vi "Untitled 22.vi"() -> ()   [LabVIEW 2010]
uses:
  <vilib>/NXT/Block Support/NXT_InputPort.ctl
  <vilib>/NXT/Subs/MotorOutput.ctl
  <vilib>/NXT/Dual Mode Library/Sensors/Sonar_cm.vi
  <vilib>/NXT/Dual Mode Library/Motors/MotorOn.vi
  <vilib>/NXT/Dual Mode Library/Motors/MotorReverse.vi
  <vilib>/NXT/Dual Mode Library/Waits/Wait_Num.vi
panel:
  in  "Time (1 sec) 2":sgl=1.0 caption="Time (1 sec)"
  in  "Time (1 sec)":sgl=1.0
  in  "Output Port (All Ports) 2":T1=3 items=["Port A", "Port B", "Port C", "All Ports"]
  in  "Power (75)":i32=75
  in  "Output Port (All Ports)":T1=3 items=["Port A", "Port B", "Port C", "All Ports"]
  in  "Port (Port 4)":T2=3 items=["Port 1", "Port 2", "Port 3", "Port 4"]
  in  "stop":bool
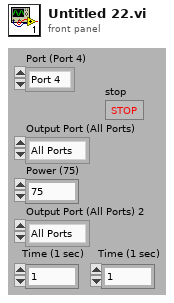
[diagram p1: front panel]
types:
  T1 = typedef "MotorOutput.ctl" = u8
  T2 = typedef "NXT_InputPort.ctl" = u8
  T3 = typedef "LVHSConnector.ctl" = cluster{"error":errorcluster, "address":string, "NXT #":i32, "Show Error":bool, "Connection":u16}
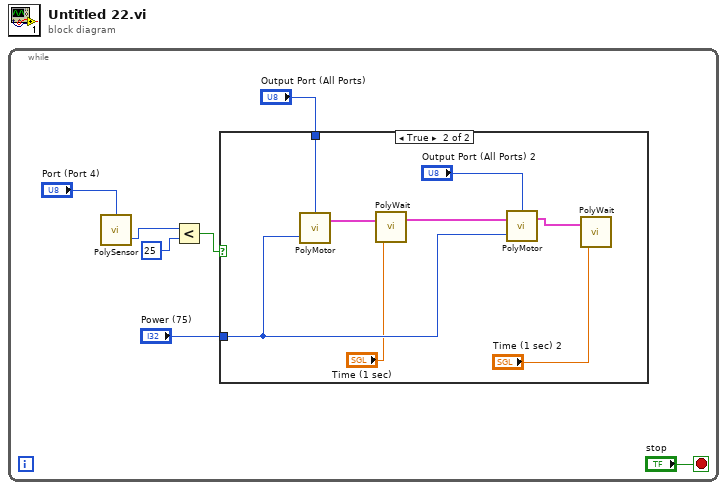
[diagram p0: block diagram]
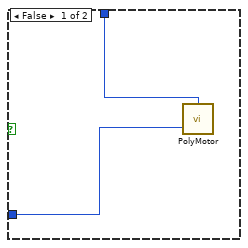
[diagram p2: hidden frame]
diagram:
  n1 = while {
    stop <- "stop" stop-if-true
    n2 = call-poly <vilib>:"PolySensor.vi"("Port (Port 4)"="Port (Port 4)") -> ("Distance (cm)"=w4:i16)  [unwired: 2 in, 1 out]
    n3 = Less?(x=w4, y=i16 25) -> (x < y?=w5:bool)
    n4 = case shown="True" w5 {
      tunnel: "Output Port (All Ports)" -> [w9 w17]
      tunnel: "Power (75)" -> [w8 w12]
      frame False {
        n5 = call-poly <vilib>:"PolyMotor.vi"("Power (75)"=w8, "Output Port (All Ports)"=w9) -> ()  [unwired: 2 in, 1 out]
      }
      frame True {
        n6 = call-poly <vilib>:"PolyMotor.vi"("Power (75)"=w12, "Output Port (All Ports)"=w17) -> ("NXT"=w16:T3)  [unwired: 2 in]
        n7 = call-poly <vilib>:"PolyWait.vi"("Time (1 sec)"="Time (1 sec)", "NXT"=w16) -> ("NXT"=w15:T3)  [unwired: 2 in]
        n8 = call-poly <vilib>:"PolyMotor.vi"("Power (75)"=w12, "NXT"=w15, "Output Port (All Ports)"="Output Port (All Ports) 2") -> ("NXT"=w14:T3)  [unwired: 1 in]
        n9 = call-poly <vilib>:"PolyWait.vi"("Time (1 sec)"="Time (1 sec) 2", "NXT"=w14) -> ()  [unwired: 2 in, 1 out]
      }
    }
  }
